vi "Ramp Segment.vi"(6 "Unit":T4, 8 "error in":errorcluster, 9 "Temperature setpoint":dbl min=0.0 max=1000.0 format="%#.1f", 10 "Ramp rate":dbl format="%#_13g", 11 "Mercury Reference In":T1) -> (0 "error out":errorcluster, 3 "Mercury Reference Out":T1)   [LabVIEW 2015, in "Mercury iXX.lvlib"]
uses:
  <instrlib>/Mercury iXX/Mercury iXX.lvlib
  <instrlib>/Mercury iXX/Public/Controls/Mercury Reference.ctl
  <instrlib>/Mercury iXX/Public/Controls/Comms Transport Layer.ctl
  <instrlib>/Mercury iXX/Private/Controls/Query Dynamic Reference.ctl
  <instrlib>/Mercury iXX/Public/Controls/Unit String.ctl
  <instrlib>/Mercury iXX/Public/Libraries/Control Loop.lvlib
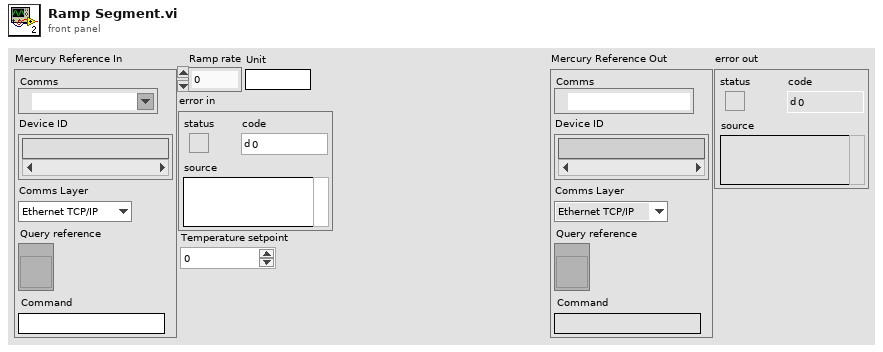
[diagram p1: front panel]
types:
  T1 = typedef "Mercury iXX.lvlib/Mercury Reference.ctl" = cluster{"Comms":refnum<visa-resource-name>, "Device ID":string[], "Comms Layer":T2, "Command":string, "Query reference":T3}
  T2 = typedef "Mercury iXX.lvlib/Comms Transport Layer.ctl" = enum16{"Ethernet TCP/IP", "USB", "ISOBus - RS-232", "GPIB"}
  T3 = typedef "Mercury iXX.lvlib/Query Dynamic Reference.ctl" = refnum<vi>
  T4 = typedef "Mercury iXX.lvlib/Unit String.ctl" = string
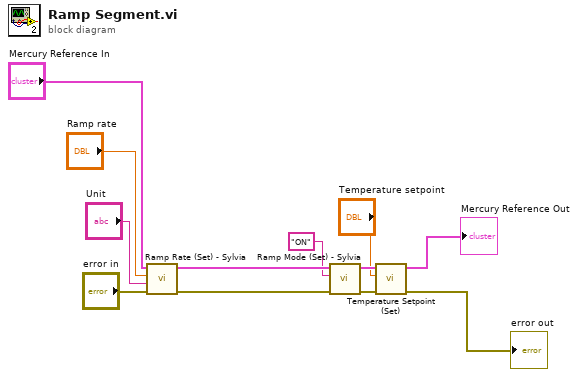
[diagram p0: block diagram]
diagram:
  n1 = call <instrlib>:"Ramp Rate (Set) - Sylvia.vi"("error in"="error in", "Unit"="Unit", "Ramp rate"="Ramp rate", "Mercury Reference In"="Mercury Reference In") -> ("error out"=w7:errorcluster, "Mercury Reference Out"=w8:T1)  [unwired: 4 in, 2 out]
  n2 = call <instrlib>:"Ramp Mode (Set) - Sylvia.vi"("error in"=w7, "Ramp Mode"="ON", "Mercury Reference In"=w8) -> ("error out"=w5:errorcluster, "Mercury Reference Out"=w4:T1)  [unwired: 5 in, 2 out]
  n3 = call <instrlib>:"Temperature Setpoint (Set).vi"("error in"=w5, "Temperature setpoint"="Temperature setpoint", "Mercury Reference In"=w4) -> ("error out"=→"error out":errorcluster, "Mercury Reference Out"=→"Mercury Reference Out":T1)  [unwired: 5 in, 2 out]
